vi "P4CMDSub UsersString to UsersList.vi"(1 "users string":string) -> (0 "users list":string[][](array[string]))   [LabVIEW 2020, in "NI_SCC_P4CMD.lvlib"]
uses:
  <vilib>/SourceControl/Providers/P4CMD/NI_SCC_P4CMD.lvlib
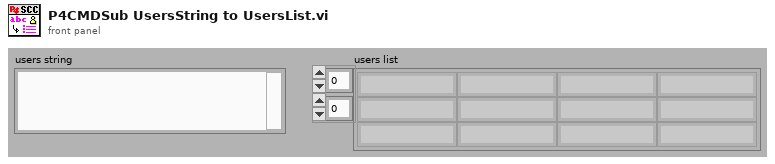
[diagram p1: front panel]
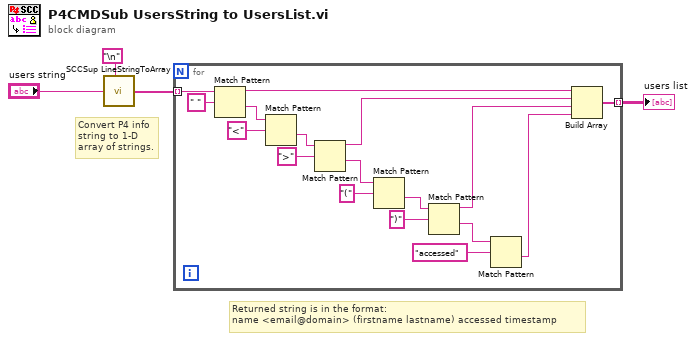
[diagram p0: block diagram]
diagram:
  # "Convert P4 info string to 1-D array of strings."
  # "Returned string is in the format:\nname <email@domain> (firstname lastname) accessed timestamp"
  n1 = call <vilib>:"SCCSup LineStringToArray.vi"("delimiter (Tab)"="\n", "line string"="users string") -> ("line array"=w1:string[])  [unwired: 7 in]
  n2 = for {
    tunnel: w1 -> [w21] mode=indexing
    tunnel: [w20] -> w4 mode=indexing
    n3 = Match Pattern(string=w21, regular expression=" ") -> (before substring=w19:string, after substring=w16:string)  [unwired: 1 in, 2 out]
    n4 = Match Pattern(string=w16, regular expression="<") -> (after substring=w14:string)  [unwired: 1 in, 3 out]
    n5 = Match Pattern(string=w14, regular expression=">") -> (before substring=w13:string, after substring=w9:string)  [unwired: 1 in, 2 out]
    n6 = Match Pattern(string=w9, regular expression="(") -> (after substring=w12:string)  [unwired: 1 in, 3 out]
    n7 = Match Pattern(string=w12, regular expression=")") -> (before substring=w8:string, after substring=w6:string)  [unwired: 1 in, 2 out]
    n8 = Match Pattern(string=w6, regular expression="accessed") -> (after substring=w5:string)  [unwired: 1 in, 3 out]
    n9 = Build Array(w19, w13, w8, w5) -> (w20:string[])
  }
  "users list" <- w4
